vi "Export Device Footprint.vi"(8 "error in (no error)":errorcluster, 10 "Destination (\"c:\\temp\\DeviceFootprint.xml\")":path=path "c:/temp/DeviceFootprint.xml", 11 "VISA resource name":refnum<visa-resource-name>="rscmx") -> (0 "error out":errorcluster, 3 "VISA resource name out":refnum<visa-resource-name>="rscmx")   [LabVIEW 2015, in "Rohde&Schwarz CMXP Base.lvlib"]
doc: "Generates an XML file with footprint information about the instrument.\n\nAttribute:\n-\n\nRemote-control command:\nSYSTem:DFPRint?"
uses:
  <instrlib>/Rohde&Schwarz CMXP Base/Rohde&Schwarz CMXP Base.lvlib
  <instrlib>/Rohde&Schwarz CMXP Base/Private/rsidr_core.llb/rsidr_core.lvlib
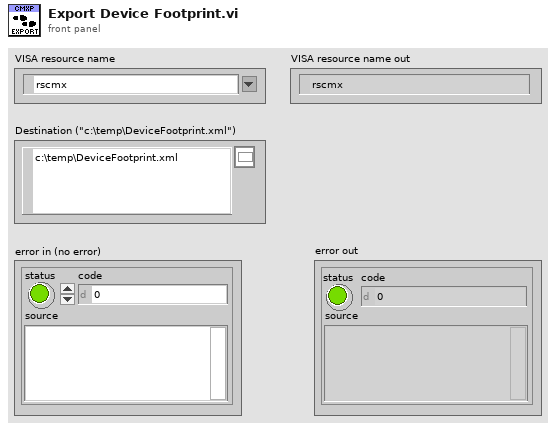
[diagram p1: front panel]
types:
  T1 = typedef "Rohde&Schwarz CMXP Base.lvlib/rsidr_core.lvlib/type_Attribute.ctl" = cluster{"Identifier":string, "Descriptive Name":string, "Data Type":T2, "Command":string, "Access":T3, "Range Table":string, "Read Callback":string, "Write Callback":string, "Supported Models":string, "Instrument Options":string, "Index":i32, "OPC Wait":bool, "No Status Check":bool, "Cache Only":bool}
  T2 = typedef "Rohde&Schwarz CMXP Base.lvlib/rsidr_core.lvlib/type_Attribute_Data_Type.ctl" = enum16{"Integer 32", "Double", "String", "Boolean", "None", "Integer 64", "RawString"}
  T3 = typedef "Rohde&Schwarz CMXP Base.lvlib/rsidr_core.lvlib/type_ReadWriteAccess.ctl" = enum16{"Read Only", "Write Only", "Read/Write"}
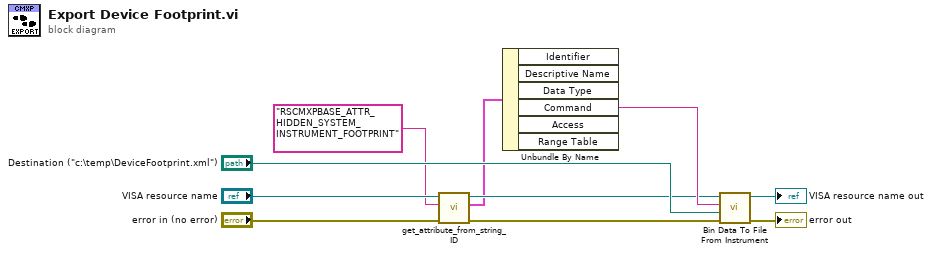
[diagram p0: block diagram]
diagram:
  n1 = call <instrlib>:"get_attribute_from_string_ID.vi"("error in"="error in (no error)", "Attribute ID in"="RSCMXPBASE_ATTR_HIDDEN_SYSTEM_INSTRUMENT_FOOTPRINT", "VISA resource name"="VISA resource name") -> ("error out"=w4:errorcluster, "Attribute out"=w1:T1, "VISA resource name out"=w5:refnum<visa-resource-name>)  [unwired: 6 in]
  n2 = Unbundle By Name(w1) -> ("Command"=w7:string)  [unwired: 5 out]
  n3 = call <instrlib>:"Bin Data To File From Instrument.vi"("error in (no error)"=w4, "Target PC File"="Destination (\"c:\\temp\\DeviceFootprint.xml\")", "Query (\"\")"=w7, "VISA resource name"=w5) -> ("error out"=→"error out":errorcluster, "VISA resource name out"=→"VISA resource name out":refnum<visa-resource-name>)  [unwired: 6 in]
